vi "Disobeying_Graph_ScalesMODCA1.vi"() -> ()   [LabVIEW 2012]
panel:
  out "Final [i]":i32
  out "XScale\nActual\nIncrement":dbl
  out "OK?":bool
  out "YScale Increment":dbl
  out "YScale Max":dbl
  out "YScale Min":dbl
  out "XScale Min":dbl
  out "XScaleMax":dbl
  out "XScale Increment":dbl
  out "rawMS":cluster{dbl[], dbl[]}(graph) caption="Current Mass Spectrum"
  # "FOR loop terminates early even though the x-increment should be invariant for the duration of the run\n(final [i] alternates between 0 and 7 in successive runs)"
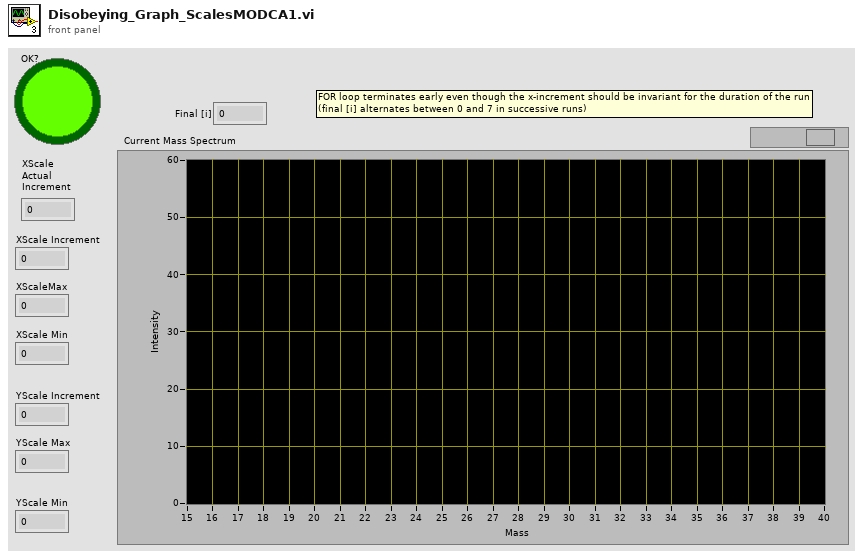
[diagram p1: front panel]
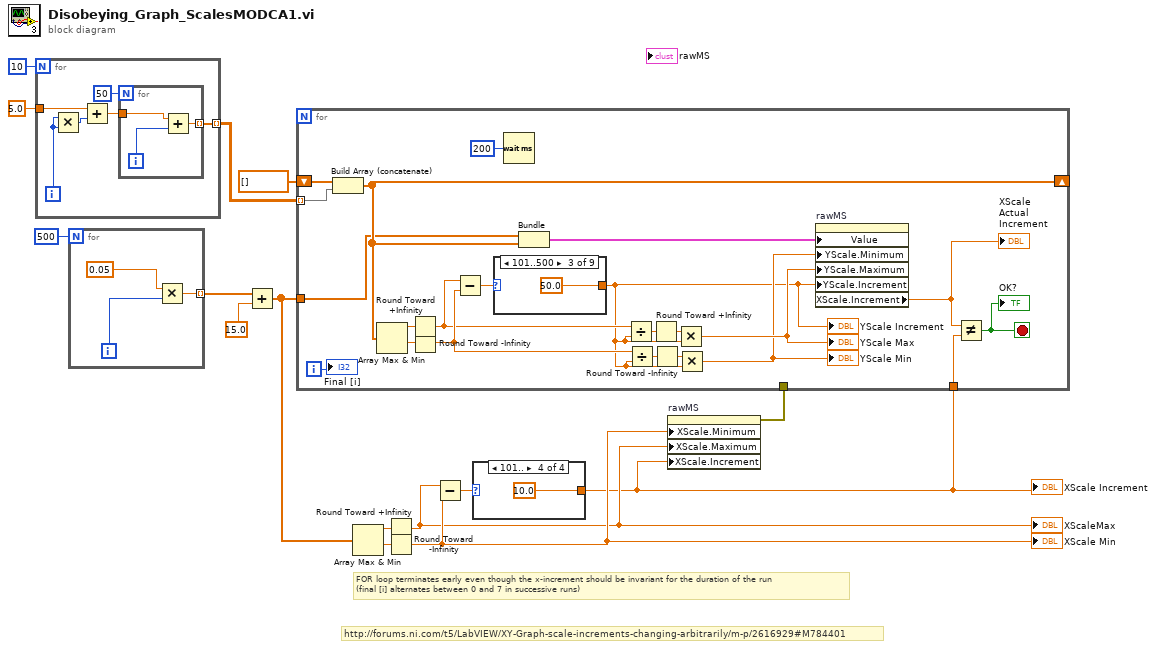
[diagram p0: block diagram]
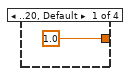
[diagram p2: hidden frame]
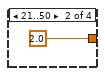
[diagram p3: hidden frame]
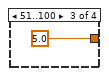
[diagram p4: hidden frame]
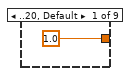
[diagram p5: hidden frame]
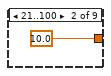
[diagram p6: hidden frame]
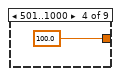
[diagram p7: hidden frame]
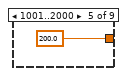
[diagram p8: hidden frame]
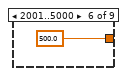
[diagram p9: hidden frame]
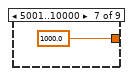
[diagram p10: hidden frame]
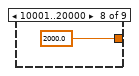
[diagram p11: hidden frame]
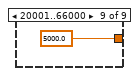
[diagram p12: hidden frame]
diagram:
  # "FOR loop terminates early even though the x-increment should be invariant for the duration of the run\n(final [i] alternates between 0 and 7 in successive runs)"
  # "http://forums.ni.com/t5/LabVIEW/XY-Graph-scale-increments-changing-arbitrarily/m-p/2616929#M784401"
  n1 = for {
    N: 10 -> [_]
    tunnel: 5.0 -> [w20]
    tunnel: [w18] -> w12 mode=indexing
    i -> [w16]
    n2 = Multiply(x=w16, y=w16) -> (x*y=w17:i32)
    n3 = Add(x=w20, y=w17) -> (x+y=w19:dbl)
    n4 = for {
      N: 50 -> [_]
      tunnel: w19 -> [w24]
      tunnel: [w23] -> w18 mode=indexing
      i -> [w22]
      n5 = Add(x=w24, y=w22) -> (x+y=w23:dbl)
    }
  }
  n6 = for {
    N: 500 -> [_]
    tunnel: [w25] -> w10 mode=indexing
    i -> [w27]
    n7 = Multiply(x=0.05, y=w27) -> (x*y=w25:dbl)
  }
  n8 = Add(x=w10, y=15.0) -> (x+y=w5:dbl[])
  n9 = Array Max & Min(array=w5) -> (max value=w8:dbl, min value=w7:dbl)  [unwired: 2 out]
  n10 = Round Toward +Infinity(x=w8) -> (ceil(x): smallest int >= x=w3:dbl)
  "XScaleMax" <- w3
  n11 = Round Toward -Infinity(1:w7) -> (0:w4:dbl)
  "XScale Min" <- w4
  n12 = Subtract(x=w3, y=w4) -> (x-y=w6:dbl)
  n13 = case shown="101.." w6 {
    tunnel: [1.0 2.0 5.0 10.0] -> w2
    frame ..20, Default {
    }
    frame 21..50 {
    }
    frame 51..100 {
    }
    frame 101.. {
    }
  }
  "XScale Increment" <- w2
  n14 = property on="rawMS" class="XYGraph (strict)"("XScale.Minimum"=w4, "XScale.Maximum"=w3, "XScale.Increment"=w2) -> (error out=w1:errorcluster)  [unwired: 2 in, 1 out]
  n15 = for {
    tunnel: w5 -> [w37]
    shift-right: [w38] -> _
    shift-left: dbl[] [] -> [w53]
    tunnel: w12 -> [w52] mode=indexing
    tunnel: w2 -> [w33]
    tunnel: w1 -> [_]
    i -> [w32]
    stop <- w36 stop-if-true
    n16 = Build Array (concatenate)(w53, w52) -> (w38:dbl[])
    n17 = Array Max & Min(array=w38) -> (max value=w42:dbl, min value=w43:dbl)  [unwired: 2 out]
    n18 = Round Toward +Infinity(x=w42) -> (ceil(x): smallest int >= x=w47:dbl)
    n19 = Round Toward -Infinity(1:w43) -> (0:w50:dbl)
    n20 = Subtract(x=w47, y=w50) -> (x-y=w44:dbl)
    n21 = case shown="101..500" w44 {
      tunnel: [1.0 10.0 50.0 100.0 200.0 500.0 1000.0 2000.0 5000.0] -> w39
      frame ..20, Default {
      }
      frame 21..100 {
      }
      frame 101..500 {
      }
      frame 501..1000 {
      }
      frame 1001..2000 {
      }
      frame 2001..5000 {
      }
      frame 5001..10000 {
      }
      frame 10001..20000 {
      }
      frame 20001..66000 {
      }
    }
    "YScale Increment" <- w39
    n22 = Wait (ms)(milliseconds to wait=u32 200) -> ()  [unwired: 1 out]
    n23 = Bundle(w37, w38) -> (w34:cluster{dbl[], dbl[]})  [unwired: 1 in]
    n24 = Divide(x=w47, y=w39) -> (x/y=w45:dbl)
    n25 = Divide(x=w50, y=w39) -> (x/y=w48:dbl)
    n26 = Round Toward +Infinity(x=w45) -> (ceil(x): smallest int >= x=w46:dbl)
    n27 = Round Toward -Infinity(1:w48) -> (0:w49:dbl)
    n28 = Multiply(x=w46, y=w39) -> (x*y=w41:dbl)
    "YScale Max" <- w41
    n29 = Multiply(x=w49, y=w39) -> (x*y=w40:dbl)
    "YScale Min" <- w40
    n30 = property on="rawMS" class="XYGraph (strict)"("Value"=w34, "YScale.Minimum"=w40, "YScale.Maximum"=w41, "YScale.Increment"=w39) -> ("XScale.Increment"=w35:dbl)  [unwired: 2 in, 2 out]
    "XScale\nActual\nIncrement" <- w35
    n31 = Not Equal?(x=w35, y=w33) -> (x != y?=w36:bool)
    "OK?" <- w36
    "Final [i]" <- w32
  }
